vi "Intra-Move Items.vi"(4 "indent":i32, 6 "Insertion index":i32, 8 "error in (no error)":errorcluster, 9 "Copy?":bool, 10 "Indices to move":i32[](array[numeric]), 11 "BetterTreeHandle in":refnum<class "BetterTreeHandle.lvclass">) -> (0 "error out":errorcluster, 3 "BetterTreeHandle out":refnum<class "BetterTreeHandle.lvclass">)   [LabVIEW 2020, in "BetterDragAndDrop.lvlib" / "BetterTreeHandle.lvclass"]
uses:
  BetterTreeHandle.lvclass
  C:/Code/GITHUB/BetterDragAndDrop/Source/Classes/BetterHandle/BetterHandle.lvclass
  BetterHandle/BetterHandle.lvclass/BetterHandle.ctl
  BetterTreeHandle.lvclass/BetterTreeHandle.ctl
  a15b403c-ceb4-457f-84d7-a210678db844.vi
  6ed20b05-8fce-4e42-93d8-9171bfb054d1.vi
  a15b403c-ceb4-457f-84d7-a210678db844.vi/bb9b305c-0eb3-4e25-bff2-b466a4ea47c4.vi
  6ed20b05-8fce-4e42-93d8-9171bfb054d1.vi/bb9b305c-0eb3-4e25-bff2-b466a4ea47c4.vi
  BetterTreeItem/SubVIs/ReAnchor Steps POLY.vi
  BetterTreeItem/SubVIs/Re-Anchor steps TreeItemObjs.vi
  BetterTreeItem/SubVIs/Re-Anchor steps TreeItem.vi
  BetterHandle/BetterHandle.lvclass
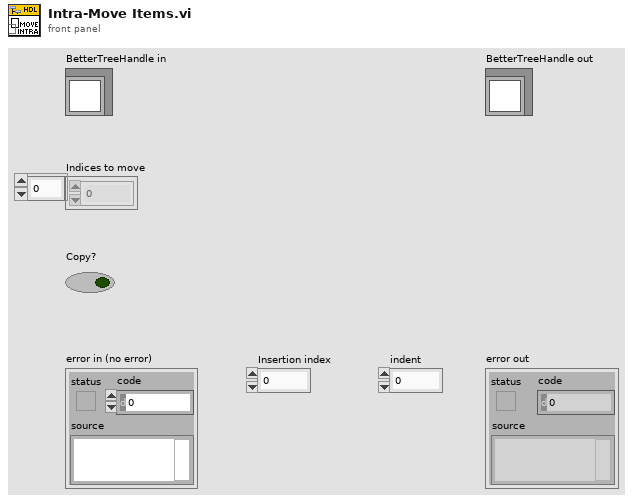
[diagram p1: front panel]
types:
  T1 = typedef "BetterDragAndDrop.lvlib/BetterTreeHandle.lvclass/TreeItem.ctl" = cluster{"Left Cell String":string, "Child Text":string[], "Child Tag":string, "Item Indent":i32, "Child Only?":bool, "Glyph Index":i32, "Font Color":u32}
  T2 = typedef "BetterDragAndDrop.lvlib/BetterTreeHandle.lvclass/Tree Move Indices.ctl" = cluster{"Parent Index":i32, "Children indices":i32[]}
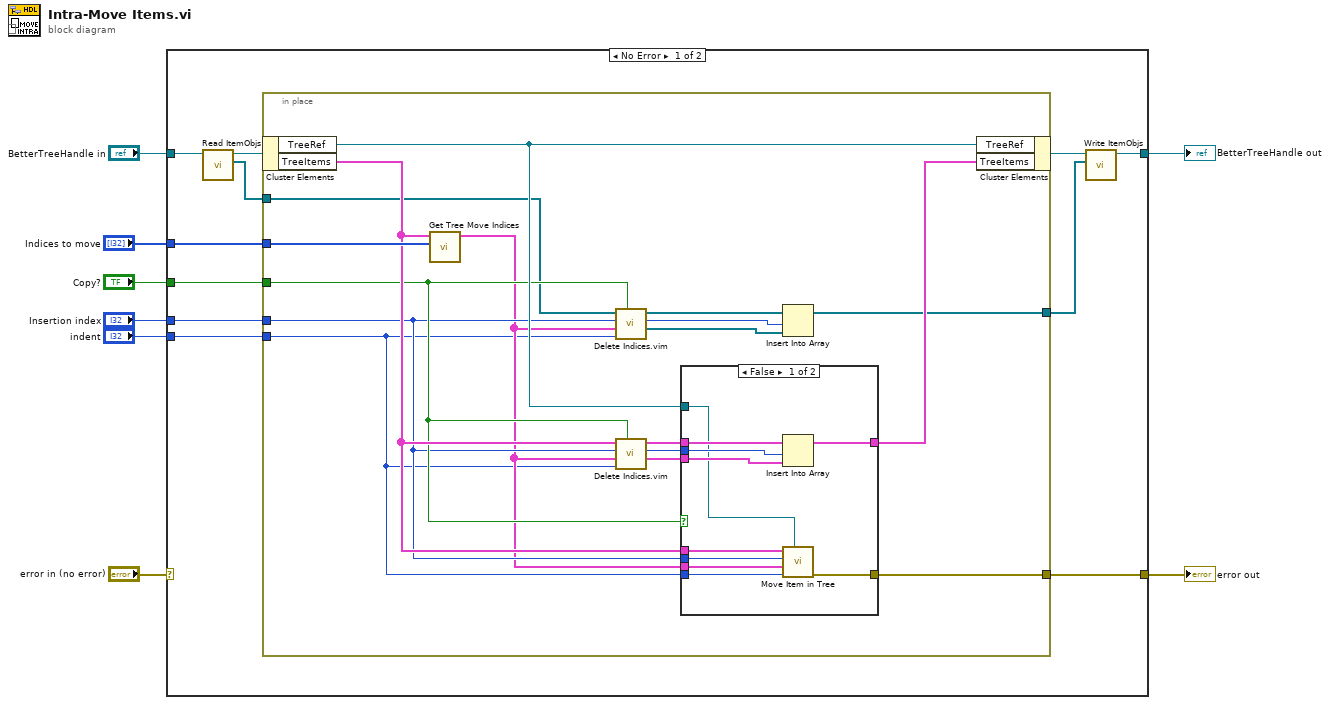
[diagram p0: block diagram]
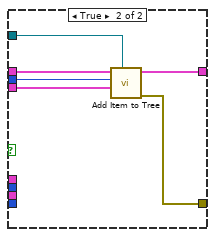
[diagram p2: hidden frame]
diagram:
  n1 = case shown="No Error" "error in (no error)" {
    selector: "error in (no error)" -> [_ w54]
    tunnel: "indent" -> [w19 _]
    tunnel: "Insertion index" -> [w18 _]
    tunnel: "Indices to move" -> [w17 _]
    tunnel: "Copy?" -> [w16 _]
    tunnel: "BetterTreeHandle in" -> [w14 w53]
    tunnel: [w10 w53] -> w3
    tunnel: [w15 w54] -> w2
    frame No Error {
      n2 = call "Read ItemObjs.vi"("BetterHandle in"=w14) -> ("ItemObjs"=w12:refnum<class "BetterItem.lvclass">[], "BetterHandle out"=w13:refnum<class "BetterTreeHandle.lvclass">)  [unwired: 9 in]
      n3 = in-place {
        in-place-border: w19 -> [w30]
        in-place-border: w18 -> [w32]
        in-place-border: w17 -> [w36]
        in-place-border: w16 -> [w33]
        in-place-border: [w22] -> w15
        in-place-border: w12 -> [w21]
        in-place-border: [w20] -> w9
        n4 = in-place-cluster #1(w13) -> ("TreeRef"=w35:refnum<vi>, "TreeItems"=w34:T1[])
        n5 = call "Get Tree Move Indices.vi"("Selected Indices"=w36, "TreeItems"=w34) -> ("Tree Move Indices"=w31:T2[])  [unwired: 9 in]
        n6 = call "Delete Indices.vim"("Copy?"=w33, "indent"=w30, "Tree Move Indices"=w31, "Insertion index"=w32, "TreeItems"=w21) -> ("elements to be inserted"=w28:refnum<class "BetterItem.lvclass">[], "new insertion index"=w27:i32, "TreeItems"=w29:refnum<class "BetterItem.lvclass">[])  [unwired: 4 in]
        n7 = call "Delete Indices.vim"("Copy?"=w33, "indent"=w30, "Tree Move Indices"=w31, "Insertion index"=w32, "TreeItems"=w34) -> ("elements to be inserted"=w26:T1[], "new insertion index"=w24:i32, "TreeItems"=w25:T1[])  [unwired: 4 in]
        n8 = case shown="False" w33 {
          tunnel: w35 -> [w37 w47]
          tunnel: [w46 w48] -> w22
          tunnel: w34 -> [w45 _]
          tunnel: w31 -> [w44 _]
          tunnel: w32 -> [w43 _]
          tunnel: w30 -> [w42 _]
          tunnel: w26 -> [w39 w52]
          tunnel: w25 -> [w41 w51]
          tunnel: w24 -> [w40 w50]
          tunnel: [w38 w49] -> w23
          frame False {
            n9 = Insert Into Array(array=w41, index=w40, new element=w39) -> (w38:T1[])
            n10 = call "Move Item in Tree.vi"("Tree ref"=w37, "Insertion indent"=w42, "Tree Move Indices"=w44, "Insertion index"=w43, "TreeItems (current)"=w45) -> ("error out"=w46:errorcluster)  [unwired: 6 in]
          }
          frame True {
            n11 = call "Add Item to Tree.vi"("Tree ref"=w47, "TreeItems (to add)"=w52, "Insertion index"=w50, "TreeItems (current)"=w51) -> ("error out"=w48:errorcluster, "TreeItems (added)"=w49:T1[])  [unwired: 6 in]
          }
        }
        n12 = Insert Into Array(array=w29, index=w27, new element=w28) -> (w20:refnum<class "BetterItem.lvclass">[])
        n13 = in-place-cluster #1("TreeRef"=w35, "TreeItems"=w23) -> (w11:refnum<class "BetterTreeHandle.lvclass">)
      }
      n14 = call "Write ItemObjs.vi"("ItemObjs"=w9, "BetterHandle in"=w11) -> ("BetterHandle out"=w10:refnum<class "BetterTreeHandle.lvclass">)  [unwired: 9 in]
    }
    frame Error {
    }
  }
  "error out" <- w2
  "BetterTreeHandle out" <- w3
